vi "DFD 2-Band Filter Bank Decomposition with State (Array).vi"(6 "state in":cluster{"state ":dbl[]}[](array[cluster]), 8 "error in (no error)":errorcluster, 9 "init? (F)":bool, 10 "analysis bank":T1={"mBank_Filters"=[], " mBank_#Bands"=2, "mBank_ProcMethod"=enum."General", "mBank_Coeffs"=[], "mBank_Gain"=1.0, "mBank_Type"=0} {"mBank_Type" items=["Uniform", "Non-Uniform"]; "mBank_Filters"."mMRate_SumWl" min=1 max=32 step=1; "mBank_Filters"."mMRate_InputIwl" min=1 max=32 step=1; "mBank_Filters"."mMRate_GainWl" min=1 max=32 step=1; "mBank_Filters"."mMRate_OutputWl" min=1 max=32 step=1; "mBank_Filters"."mMRate_InputWl" min=1 max=32 step=1; "mBank_Filters"."mMRate_CoefWl" min=1 max=32 step=1; "mBank_Filters"."mMRate_Mode" items=["Default"=-1, "No Rate Change"=0, "Interpolation"=1, "Decimation"=2, "Interpolated"=3, "Rational"=4]}, 11 "x":dbl[](array[numeric]) format="%.2f") -> (0 "error out":errorcluster, 2 "highpass band":dbl[](array[numeric]), 3 "lowpass band":dbl[](array[numeric]), 4 "state out":cluster{"state ":dbl[]}[](array[cluster]))   [LabVIEW 2017, in "NI_DigFilter_FilterBank.lvlib"]
doc: "Filters the input sequence <B>x</B> using a 2-band analysis bank specified by <B>analysis bank</B>. You must specify the most recent internal input states <B>state in</B> to get the correct output. \n\n<B>state out</B> contains the most recent internal output states, which can be used as <B>state in</B> for next call to this VI if you want to process the data continuously.\n\nYou can call the VIs in <B>Filter Bank Design</B> sub-palette to design a filter bank."
uses:
  <vilib>/addons/Digital Filter Design/NI_DigFilter_FilterBank.lvlib
  <vilib>/addons/Digital Filter Design/FilterBank.llb/Object/DFD Bank Obj.ctl
  <vilib>/addons/Digital Filter Design/_Objects.llb/DFD Multirate Filter Obj.ctl
  <vilib>/addons/Digital Filter Design/_Objects.llb/DFD Multirate Mode.ctl
  <vilib>/addons/Digital Filter Design/_Objects.llb/DFD Coef Norm Type.ctl
  <vilib>/addons/Digital Filter Design/_Objects.llb/DFD Round-off Mode.ctl
  <vilib>/addons/Digital Filter Design/_Objects.llb/DFD FXP MRate Multiply Mode.ctl
  <vilib>/addons/Digital Filter Design/FilterBank.llb/Object/DFD Filter Bank Processing Method.ctl
  <vilib>/addons/Digital Filter Design/FilterBank.llb/Object/DFD Filter Bank Type.ctl
  <vilib>/addons/Digital Filter Design/NI_DigFilterLicensed.lvlib
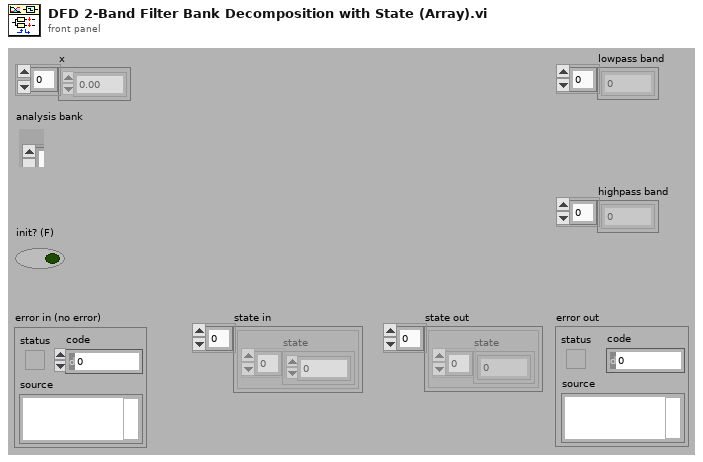
[diagram p1: front panel]
types:
  T1 = typedef "NI_DigFilter_FilterBank.lvlib/DFD Bank Obj.ctl" = cluster{"mBank_Filters":T2[], " mBank_#Bands":i32, "mBank_ProcMethod":T7, "mBank_Coeffs":dbl[], "mBank_Gain":dbl, "mBank_Type":T8}
  T2 = typedef "NI_DigFilterLicensed.lvlib/DFD Multirate Filter Obj.ctl" = cluster{"mMRate_Structure":enum16{"CIC", "FIR", "IIR", "Lattice"}, "mMRate_Mode":T3, "mMRate_Factor":i32, "mMRate_FIRParams":cluster{"mMRate_FIR_H":dbl[], "mMRate_FIR_IsNyquist?":bool, "mMRate_FIR_IsSymmetric?":bool}, "mMRate_CICParams":cluster{"mMRate_CIC_#Stage":i32, "mMRate_CIC_Lag":i32, "mMRate_CIC_Type":enum16{"Lowpass", "Highpass"}}, "mMRate_Order":i32, "mMRate_Version":string, "mMRate_Comments":string, "mMRate_RationalFactor":cluster{"mMRate_L":i32, "mMRate_M":i32}, "mMRate_Fs":dbl, "mMRate_Quantized?":bool, "mMRate_QFilterGain":dbl, "mMRate_CoefWl":i16, "mMRate_Scaling":cluster{"mMRate_ScaleByPowerOf2?":bool, "mMRate_ScaleType":T4}, "mMRate_InputWl":i16, "mMRate_OutputWl":i16, "mMRate_OutputMode":T5, "mMRate_MultMode":T6, "mMRate_BitPruning":bool, "mMRate_GainWl":i16, "mMRate_OutputFwl":i16, "mMRate_SumIwl":i16, "mMRate_InputIwl ":i16, "mMRate_SumWl":i16, "mMRate_CoefIwl":i16}
  T3 = typedef "NI_DigFilterLicensed.lvlib/DFD Multirate Mode.ctl" = i16
  T4 = typedef "NI_DigFilterLicensed.lvlib/DFD Coef Norm Type.ctl" = enum16{"No Norm", "Time Domain 1-Norm", "Time Domain 2-Norm", "Time Domain Inf-Norm"}
  T5 = typedef "NI_DigFilterLicensed.lvlib/DFD Round-off Mode.ctl" = enum16{"Nearest", "Truncation"}
  T6 = typedef "NI_DigFilterLicensed.lvlib/DFD FXP MRate Multiply Mode.ctl" = enum16{"Truncated", "Full"}
  T7 = typedef "NI_DigFilter_FilterBank.lvlib/DFD Filter Bank Processing Method.ctl" = enum16{"General", "2-Band QMF Lattice", "Cosine-Modulated"}
  T8 = typedef "NI_DigFilter_FilterBank.lvlib/DFD Filter Bank Type.ctl" = u16
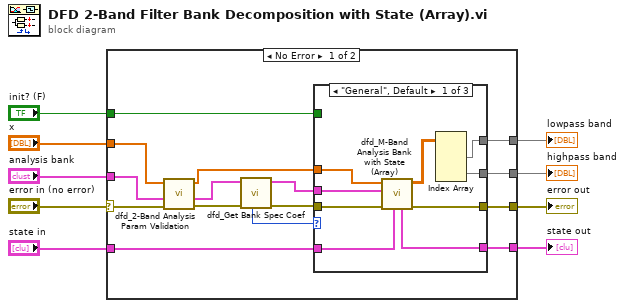
[diagram p0: block diagram]
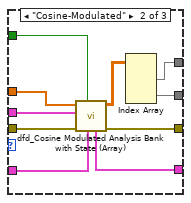
[diagram p2: hidden frame]
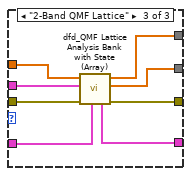
[diagram p3: hidden frame]
diagram:
  n1 = case shown="No Error" "error in (no error)" {
    selector: "error in (no error)" -> [w17 w52]
    tunnel: "analysis bank" -> [w16 _]
    tunnel: "state in" -> [w24 _]
    tunnel: "x" -> [w19 _]
    tunnel: [w23 _] -> w2
    tunnel: [w22 _] -> w8
    tunnel: [w21 _] -> w7
    tunnel: [w20 w52] -> w6
    tunnel: "init? (F)" -> [w15 _]
    frame No Error {
      n2 = call <vilib>:"dfd_2-Band Analysis Param Validation.vi"("error in (no error)"=w17, "bank"=w16, "x"=w19) -> ("error out"=w13:errorcluster, "dup bank"=w14:T1, "dup x"=w18:dbl[])  [unwired: 6 in]
      n3 = call <vilib>:"dfd_Get Bank Spec Coef.vi"("error in (no error)"=w13, "bank in"=w14) -> ("error out"=w12:errorcluster, "bank out"=w10:T1, "processing method"=w11:T7)  [unwired: 4 in, 3 out]
      n4 = case shown="\"General\", Default" w11 {
        tunnel: w24 -> [w30 w41 w47]
        tunnel: w18 -> [w32 w42 w51]
        tunnel: w12 -> [w25 w36 w50]
        tunnel: [w33 w43 w49] -> w20
        tunnel: [w31 w38 w46] -> w23
        tunnel: [w29 w40 w48] -> w22
        tunnel: [w28 w39 w45] -> w21
        tunnel: w10 -> [w26 w35 w44]
        tunnel: w15 -> [_ w34 _]
        frame "General", Default {
          n5 = call <vilib>:"dfd_M-Band Analysis Bank with State (Array).vi"("state in"=w30, "error in"=w25, "bank in"=w26, "x"=w32) -> ("error out"=w33:errorcluster, "y"=w27:dbl[][], "state out"=w31:cluster{"state ":dbl[]}[])  [unwired: 5 in]
          n6 = Index Array(array=w27) -> (element #1=w29:dbl[], element #2=w28:dbl[])  [unwired: 4 in]
        }
        frame "Cosine-Modulated" {
          n7 = call <vilib>:"dfd_Cosine Modulated Analysis Bank with State (Array).vi"("state in"=w41, "init?"=w34, "error in (no error)"=w36, "bank in"=w35, "x"=w42) -> ("error out"=w43:errorcluster, "y"=w37:dbl[][], "state out"=w38:cluster{"state ":dbl[]}[])  [unwired: 4 in]
          n8 = Index Array(array=w37) -> (element #1=w40:dbl[], element #2=w39:dbl[])  [unwired: 4 in]
        }
        frame "2-Band QMF Lattice" {
          n9 = call <vilib>:"dfd_QMF Lattice Analysis Bank with State (Array).vi"("state in"=w47, "error in (no error)"=w50, "filter bank in"=w44, "x"=w51) -> ("error out"=w49:errorcluster, "highpass channel"=w45:dbl[], "lowpass channel"=w48:dbl[], "state out"=w46:cluster{dbl[]}[])  [unwired: 4 in]
        }
      }
    }
    frame Error {
    }
  }
  "lowpass band" <- w8
  "highpass band" <- w7
  "error out" <- w6
  "state out" <- w2
